vi "receive.vi"() -> ()   [LabVIEW 2018]
uses:
  <vilib>/Instr/_visa.llb/VISA Configure Serial Port (Instr).vi
panel:
  in  "接收":bool
  in  "文件路径":path
  in  "停止":bool
  in  "VISA资源名称":refnum<visa-resource-name>
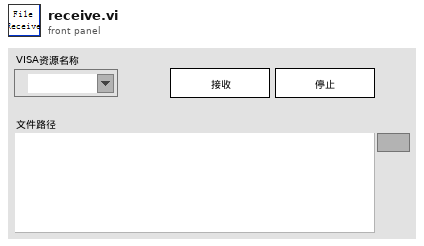
[diagram p1: front panel]
types:
  T1 = enum16{"open", "replace", "create", "open or create", "replace or create", "replace or create with confirmation"}
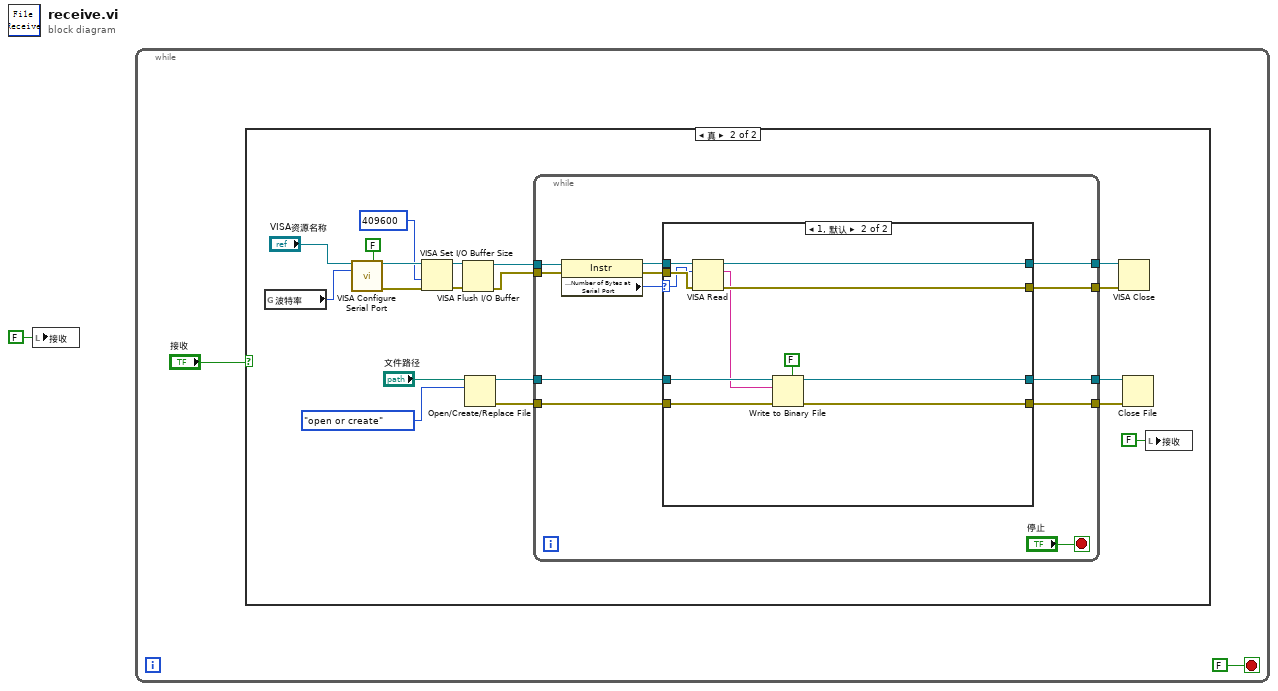
[diagram p0: block diagram]
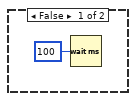
[diagram p2: hidden frame]
diagram:
  n1 = local write "接收"(FALSE ("接收")) -> ()
  n2 = while {
    stop <- FALSE stop-if-true
    n3 = case shown="真" "接收" {
      frame False {
        n4 = Wait (ms)(milliseconds to wait=u32 100 ("等待时间（毫秒）")) -> ()  [unwired: 1 out]
      }
      frame True {
        n5 = global read "全局变量.vi" "波特率"() -> (w5:u32)
        n6 = call-poly "VISA Configure Serial Port"("VISA resource name"="VISA资源名称", "Enable Termination\nChar (T)"=FALSE ("Enable Termination\nChar (T)"), "baud rate (9600)"=w5) -> ("VISA resource name out"=w15:refnum<visa-resource-name>, "error out"=w12:errorcluster)  [unwired: 11 in]
        n7 = VISA Set I/O Buffer Size(VISA resource name=w15, size (4096)=u32 409600 ("大小(4096)"), error in (no error)=w12) -> (VISA resource name out=w14:refnum<visa-resource-name>, error out=w11:errorcluster)  [unwired: 1 in]
        n8 = VISA Flush I/O Buffer(VISA resource name=w14, error in (no error)=w11) -> (VISA resource name out=w13:refnum<visa-resource-name>, error out=w10:errorcluster)  [unwired: 1 in]
        n9 = Open/Create/Replace File(file path (use dialog)="文件路径", operation (0:open)=T1."open or create" ("操作(0:open)")) -> (refnum out=w22:refnum<file>, error out=w21:errorcluster)  [unwired: 4 in, 1 out]
        n10 = while {
          tunnel: w13 -> [w35]
          tunnel: w10 -> [w34]
          tunnel: [w30] -> w17
          tunnel: [w29] -> w16
          tunnel: w22 -> [w28]
          tunnel: w21 -> [w27]
          tunnel: [w26] -> w19
          tunnel: [w25] -> w18
          stop <- "停止" stop-if-true
          n11 = property class="Instr"(reference=w35, error in=w34) -> (reference out=w33:refnum<visa-resource-name>, error out=w31:errorcluster, "Serial Settings:Number of Bytes at Serial Port"=w32:u32)
          n12 = case shown="1, 默认" w32 {
            selector: w32 -> [_ w44]
            tunnel: w33 -> [w37 w50]
            tunnel: w31 -> [w36 w46]
            tunnel: [w37 w47] -> w30
            tunnel: [w36 w45] -> w29
            tunnel: w28 -> [w39 w49]
            tunnel: w27 -> [w38 w48]
            tunnel: [w39 w43] -> w26
            tunnel: [w38 w42] -> w25
            frame 0 {
            }
            frame 1, Default {
              n13 = VISA Read(VISA resource name=w50, byte count=w44, error in (no error)=w46) -> (VISA resource name out=w47:refnum<visa-resource-name>, read buffer=w41:string, error out=w45:errorcluster)  [unwired: 1 out]
              n14 = Write to Binary File(file (use dialog)=w49, data=w41, error in=w48, 5:FALSE ("预置数组或字符串大小？ (T)")) -> (refnum out=w43:refnum<file>, error out=w42:errorcluster)  [unwired: 2 in, 1 out]
            }
          }
        }
        n15 = VISA Close(VISA resource name=w17, error in (no error)=w16) -> ()  [unwired: 1 out]
        n16 = Close File(refnum=w19, error in=w18) -> ()  [unwired: 2 out]
        n17 = local write "接收"(FALSE ("接收")) -> ()
      }
    }
  }
